vi "FlatToRichnixnet_grpc_InterfaceRefArray.vi"(5 "OutputClusterType":T1, 11 "InputCluster":T3) -> (3 "OutputCluster":T1)   [LabVIEW 2025, in "grpc-xnet_client.lvlib"]
uses:
  grpc-xnet_client.lvlib
  nixnet_grpc_InterfaceRefArray_Flat.ctl
  nidevice_grpc_Session_Flat.ctl
  nixnet_grpc_InterfaceRefArray.ctl
  nidevice_grpc_Session.ctl
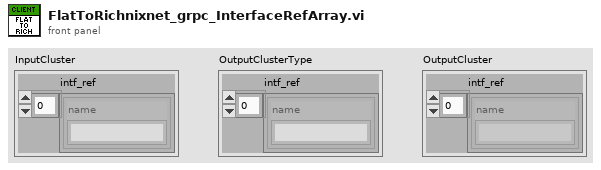
[diagram p1: front panel]
types:
  T1 = typedef "grpc-xnet_client.lvlib/nixnet_grpc_InterfaceRefArray.ctl" = cluster{"intf_ref":T2[]}
  T2 = typedef "grpc-xnet_client.lvlib/nidevice_grpc_Session.ctl" = cluster{"name":string}
  T3 = typedef "grpc-xnet_client.lvlib/nixnet_grpc_InterfaceRefArray_Flat.ctl" = cluster{"intf_ref":T4[]}
  T4 = typedef "grpc-xnet_client.lvlib/nidevice_grpc_Session_Flat.ctl" = cluster{"name":string}
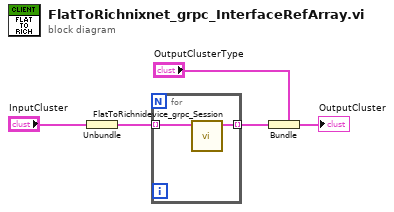
[diagram p0: block diagram]
diagram:
  n1 = Unbundle "Unbundle"("InputCluster") -> ("intf_ref"=w2:T4[])
  n2 = for {
    tunnel: w2 -> [w7] mode=indexing
    tunnel: [w6] -> w1 mode=indexing
    n3 = call "FlatToRichnidevice_grpc_Session.vi"("InputCluster"=w7) -> ("OutputCluster"=w6:T2)  [unwired: 10 in]
  }
  n4 = Bundle "Bundle"(cluster="OutputClusterType", "intf_ref"=w1) -> (→"OutputCluster":T1)
